vi "inteference -- find center V3.vi"(7 "number of points":i32, 8 "complex region":T1={"max re"=5.161869466666667e-06, "min re"=5.176843333333334e-06, "max im"=-2.467216e-05, "min im"=-0.001573233, "delta re"=0.003211203, "delta im"=0.00165815, "center re"=0.0015485608400000002, "delta  z"=0.0015530530000000002+0.0i, "center im"=0.0, "center z"=0.0+0.0i, "d im"=0.0, "d re"=0.0, "d z"=0.0+0.0i}, 9 "pond":cdb[][](array[numeric]), 10 "point sources":cdb[](array[numeric]), 11 "wave packet":cdb[][](array[numeric])) -> (2 "z (center)":cdb)   [LabVIEW 2010]
uses:
  complex region.ctl
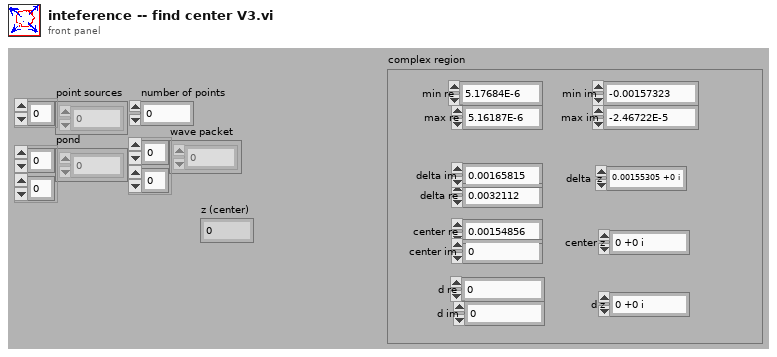
[diagram p1: front panel]
types:
  T1 = typedef "complex region.ctl" = cluster{"max re":dbl, "min re":dbl, "max im":dbl, "min im":dbl, "delta re":dbl, "delta im":dbl, "center re":dbl, "delta  z":cdb, "center im":dbl, "center z":cdb, "d im":dbl, "d re":dbl, "d z":cdb}
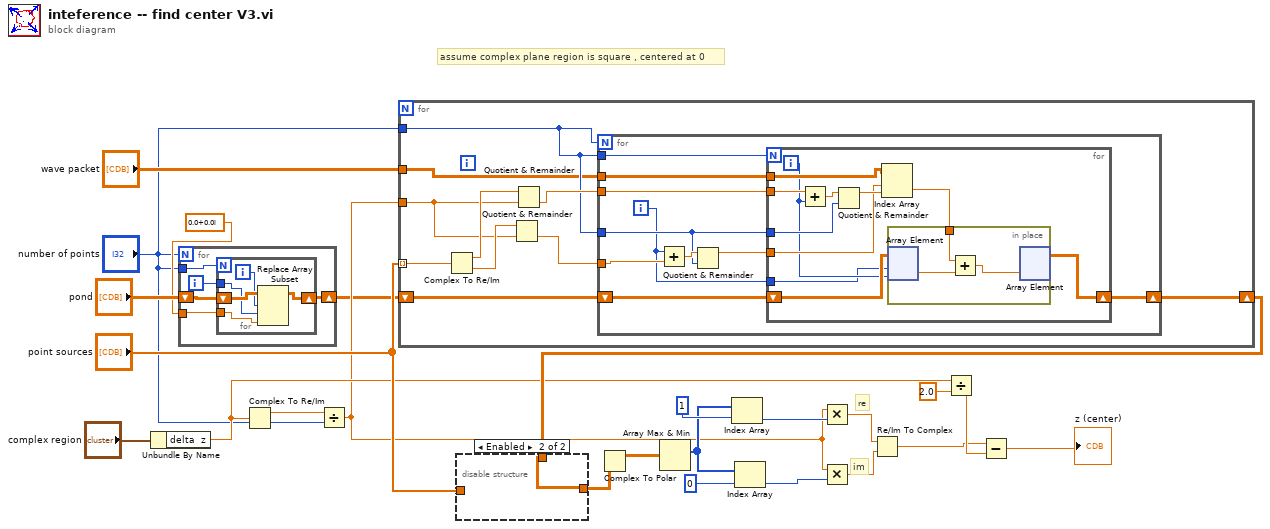
[diagram p0: block diagram]
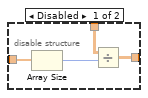
[diagram p2: hidden frame]
diagram:
  # "assume complex plane region is square , centered at 0"
  # "re"
  # "im"
  n1 = Unbundle By Name("complex region") -> ("delta  z"=w9:cdb)
  n2 = for {
    N: "number of points" -> [_]
    tunnel: cdb 0.0+0.0i -> [w28]
    shift-right: [w26] -> w2
    shift-left: "pond" -> [w29]
    tunnel: "number of points" -> [w25]
    i -> [w27]
    n3 = for {
      N: w25 -> [_]
      tunnel: w28 -> [w30]
      tunnel: w27 -> [w33]
      shift-right: [w32] -> w26
      shift-left: w29 -> [w34]
      i -> [w31]
      n4 = Replace Array Subset(array=w34, new element=w30, index (row)=w31, index (col)=w33) -> (w32:cdb[][])
    }
  }
  n5 = Complex To Re/Im(x + iy=w9) -> (x=w13:dbl)  [unwired: 1 out]
  n6 = Divide(x=w13, y="number of points") -> (x/y=w5:dbl)
  n7 = for {
    shift-right: [w35] -> w24
    shift-left: w2 -> [w36]
    tunnel: "point sources" -> [w42] mode=indexing
    tunnel: "wave packet" -> [w38]
    tunnel: w5 -> [w41]
    tunnel: "number of points" -> [w39]
    n8 = Complex To Re/Im(x + iy=w42) -> (x=w44:dbl, y=w43:dbl)
    n9 = Quotient & Remainder(x=w43, y=w41) -> (floor(x/y)=w37:dbl)  [unwired: 1 out]
    n10 = Quotient & Remainder(x=w44, y=w41) -> (floor(x/y)=w40:dbl)  [unwired: 1 out]
    n11 = for {
      N: w39 -> [_]
      tunnel: w39 -> [w54]
      tunnel: w40 -> [w53]
      tunnel: w39 -> [w49]
      tunnel: w38 -> [w52]
      tunnel: w37 -> [w50]
      shift-right: [w45] -> w35
      shift-left: w36 -> [w47]
      i -> [w46]
      n12 = Add(x=w46, y=w50) -> (x+y=w51:dbl)
      n13 = Quotient & Remainder(x=w51, y=w49) -> (x-y*floor(x/y)=w48:dbl)  [unwired: 1 out]
      n14 = for {
        N: w54 -> [_]
        tunnel: w53 -> [w65]
        tunnel: w49 -> [w63]
        tunnel: w52 -> [w62]
        tunnel: w48 -> [w60]
        shift-right: [w55] -> w45
        shift-left: w47 -> [w58]
        tunnel: w46 -> [w56]
        i -> [w57]
        n15 = Add(x=w65, y=w57) -> (x+y=w64:dbl)
        n16 = Quotient & Remainder(x=w64, y=w63) -> (x-y*floor(x/y)=w61:dbl)  [unwired: 1 out]
        n17 = Index Array(array=w62, index (row)=w60, index (col)=w61) -> (element=w59:cdb)
        n18 = in-place {
          in-place-border: w59 -> [w68]
          n19 = in-place-array #1(w58, w56, w57) -> (w67:cdb)
          n20 = Add(x=w68, y=w67) -> (x+y=w66:cdb)
          n21 = in-place-array #1(w66) -> (w55:cdb[][])  [unwired: 2 out]
        }
      }
    }
  }
  n22 = disable-structure shown="Enabled" {
    disable-tunnel: w24 -> [w72 w73]
    disable-tunnel: "point sources" -> [w70 _]
    disable-tunnel: [w69 w73] -> w18
    frame Disabled {
      n23 = Array Size(array=w70) -> (size(s)=w71:i32)
      n24 = Divide(x=w72, y=w71) -> (x/y=w69:cdb[][])
    }
    frame Enabled {
    }
  }
  n25 = Complex To Polar(r * e^(i*theta)=w18) -> (r=w17:dbl[][])  [unwired: 1 out]
  n26 = Array Max & Min(array=w17) -> (max index (indices)=w16:i32[])  [unwired: 3 out]
  n27 = Index Array(array=w16, index=1) -> (element=w15:i32)
  n28 = Index Array(array=w16, index=0) -> (element=w14:i32)
  n29 = Multiply(x=w5, y=w15) -> (x*y=w12:dbl)
  n30 = Multiply(x=w5, y=w14) -> (x*y=w11:dbl)
  n31 = Re/Im To Complex(1:w11, 2:w12) -> (0:w7:cdb)
  n32 = Divide(x=w9, y=2.0) -> (x/y=w8:cdb)
  n33 = Subtract(x=w7, y=w8) -> (x-y=→"z (center)":cdb)
